vi "MultiplyTwoMatrixes.vi"(9 "Real Matrix 2":T1, 11 "Real Matrix":T1) -> (3 "Real Matrix 3":T1)   [LabVIEW 2013]
uses:
  <vilib>/Analysis/Matrix/Datatypes/RealMatrix.ctl
  <vilib>/Analysis/Matrix/Numeric/Multiply/Multiply - RM,RM.vi
  <vilib>/Analysis/Matrix/NI_Matrix.lvlib
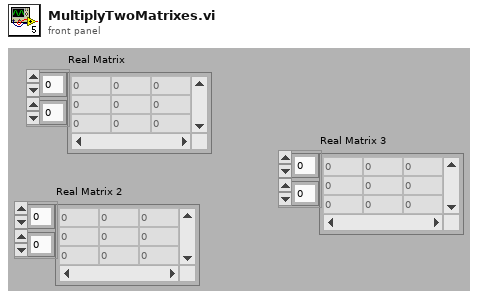
[diagram p1: front panel]
types:
  T1 = typedef "NI_Matrix.lvlib/RealMatrix.ctl" = dbl[][]
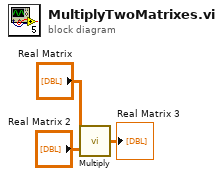
[diagram p0: block diagram]
diagram:
  n1 = call-poly <vilib>:"Multiply.vi"("Real Matrix B"="Real Matrix 2", "Real Matrix A"="Real Matrix") -> ("A * B"=→"Real Matrix 3":T1)
